vi "xy validity.vi"(9 "x input":dbl, 10 "y input":dbl) -> (3 "Validity":bool)   [LabVIEW 2020]
uses:
  Robot Global Data.vi
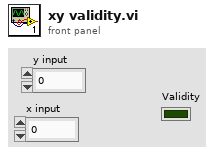
[diagram p1: front panel]
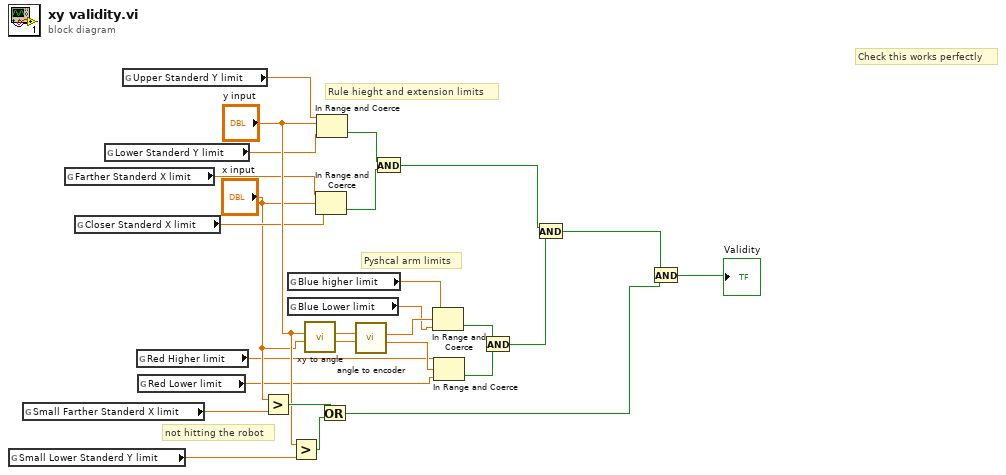
[diagram p0: block diagram]
diagram:
  # "Check this works perfectly"
  # "Pyshcal arm limits"
  # "Rule hieght and extension limits"
  # "not hitting the robot"
  n1 = global read "Robot Global Data.vi" "Small Lower Standerd Y limit"() -> (w1:dbl)
  n2 = global read "Robot Global Data.vi" "Small Farther Standerd X limit"() -> (w2:dbl)
  n3 = global read "Robot Global Data.vi" "Farther Standerd X limit"() -> (w7:dbl)
  n4 = global read "Robot Global Data.vi" "Closer Standerd X limit"() -> (w9:dbl)
  n5 = global read "Robot Global Data.vi" "Lower Standerd Y limit"() -> (w10:dbl)
  n6 = global read "Robot Global Data.vi" "Upper Standerd Y limit"() -> (w11:dbl)
  n7 = global read "Robot Global Data.vi" "Red Higher limit"() -> (w4:dbl)
  n8 = global read "Robot Global Data.vi" "Red Lower limit"() -> (w3:dbl)
  n9 = Greater?(x="x input", y=w2) -> (0:w16:bool)
  n10 = global read "Robot Global Data.vi" "Blue higher limit"() -> (w6:dbl)
  n11 = global read "Robot Global Data.vi" "Blue Lower limit"() -> (w5:dbl)
  n12 = Greater?(x="y input", y=w1) -> (0:w17:bool)
  n13 = call "xy to angle.vi"("x"="x input", "y"="y input") -> ("red angle"=w24:dbl, "Blue angle"=w25:dbl)  [unwired: 8 in]
  n14 = In Range and Coerce(upper limit=w7, x="x input", lower limit=w9) -> (In Range?=w26:bool)  [unwired: 1 out]
  n15 = In Range and Coerce(upper limit=w11, x="y input", lower limit=w10) -> (In Range?=w27:bool)  [unwired: 1 out]
  n16 = Or(x=w16, y=w17) -> (x .or. y?=w14:bool)
  n17 = call "angle to encoder.vi"("red angle"=w24, "blue angle"=w25) -> ("red encoder"=w22:dbl, "blue encoder"=w23:dbl)  [unwired: 8 in]
  n18 = And(x=w27, y=w26) -> (x .and. y?=w19:bool)
  n19 = In Range and Coerce(upper limit=w6, x=w23, lower limit=w5) -> (In Range?=w21:bool)  [unwired: 1 out]
  n20 = In Range and Coerce(upper limit=w4, x=w22, lower limit=w3) -> (In Range?=w20:bool)  [unwired: 1 out]
  n21 = And(x=w21, y=w20) -> (x .and. y?=w18:bool)
  n22 = And(x=w19, y=w18) -> (x .and. y?=w13:bool)
  n23 = And(x=w13, y=w14) -> (x .and. y?=→"Validity":bool)
